vi "GetAreaInfo.vi"(0 "TCP网络连接输入":refnum<k5>, 7 "reference":refnum<vi>, 11 "错误输入（无错误）":errorcluster) -> (8 "值":string[][](array[string]), 15 "错误输出":errorcluster)   [LabVIEW 2014]
uses:
  Global/ClientGlobalCY.vi
panel:
  out "连接的字符串":string
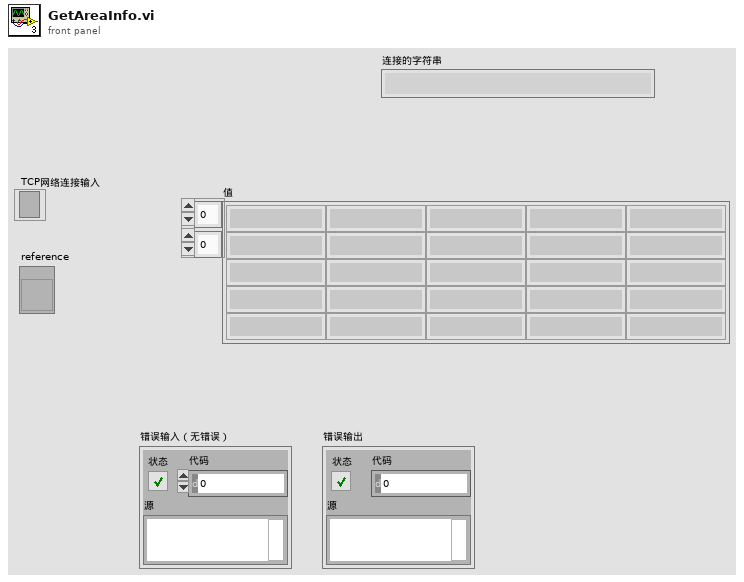
[diagram p1: front panel]
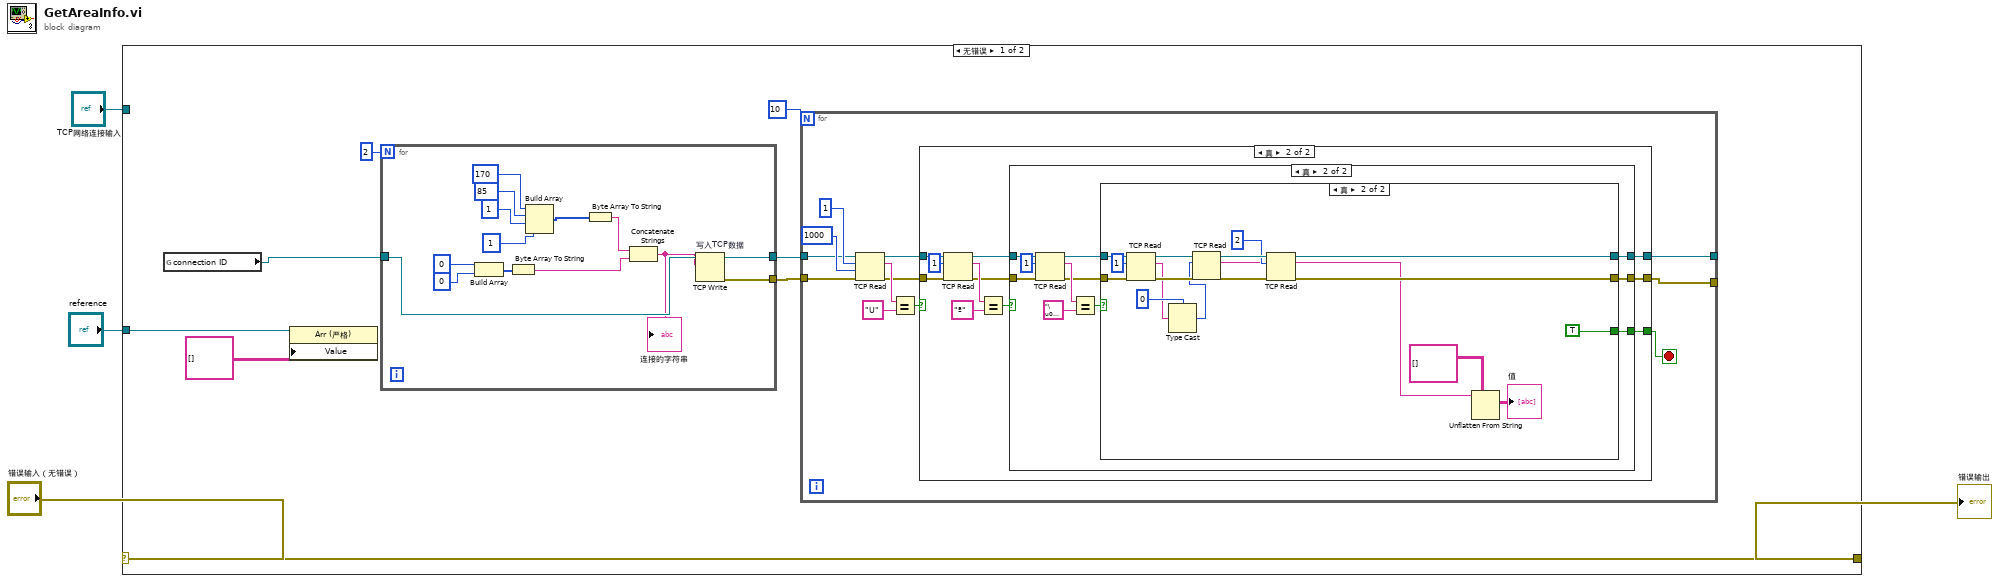
[diagram p0: block diagram]
diagram:
  n1 = case shown="无错误" "错误输入（无错误）" {
    selector: "错误输入（无错误）" -> [w12 w84]
    tunnel: [w12 w84] -> w4
    tunnel: "TCP网络连接输入" -> [_ _]
    tunnel: "reference" -> [w7 _]
    frame No Error {
      n2 = global read "ClientGlobalCY.vi" "connection ID"() -> (w5:refnum<k5>)
      n3 = property class="Arr (严格)"(reference=w7, "Value"=string[][] [] ("值")) -> ()  [unwired: 1 in, 2 out]
      n4 = for {
        N: 2 -> [_]
        tunnel: [w25] -> w10
        tunnel: w5 -> [w24]
        tunnel: [w26] -> w11
        n5 = Build Array(u8 0, u8 0) -> (w17:u8[])
        n6 = Byte Array To String(unsigned byte array=w17) -> (string=w13:string)
        n7 = Build Array(u8 170, u8 85, u8 1, u8 1) -> (w20:u8[])
        n8 = Byte Array To String(unsigned byte array=w20) -> (string=w16:string)
        n9 = Concatenate Strings(w16, w13) -> (w15:string)
        "连接的字符串" <- w15
        n10 = TCP Write "写入TCP数据"(connection ID=w24, data in=w15) -> (connection ID out=w26:refnum<k5>, error out=w25:errorcluster)  [unwired: 2 in, 1 out]
      }
      n11 = for "For循环" {
        N: 10 -> [_]
        tunnel: w11 -> [w31]
        tunnel: w10 -> [w30]
        tunnel: [w28] -> _
        tunnel: [w27] -> _
        stop <- w29 stop-if-true
        n12 = TCP Read(connection ID=w31, bytes to read=1 ("读取的字节"), error in (no error)=w30, 9:1000 ("超时毫秒(25000)")) -> (connection ID out=w34:refnum<k5>, data out=w36:string, error out=w33:errorcluster)  [unwired: 1 in]
        n13 = Equal?(x=w36, y="U") -> (x = y?=w35:bool)
        n14 = case shown="真" w35 {
          tunnel: w34 -> [w40 w48]
          tunnel: w33 -> [w39 w47]
          tunnel: [w40 w43] -> w28
          tunnel: [w39 w42] -> w27
          tunnel: [_ w41] -> w29
          frame False {
          }
          frame True {
            n15 = TCP Read(connection ID=w48, bytes to read=1 ("读取的字节"), error in (no error)=w47) -> (connection ID out=w45:refnum<k5>, data out=w49:string, error out=w44:errorcluster)  [unwired: 2 in]
            n16 = Equal?(x=w49, y="ª") -> (x = y?=w46:bool)
            n17 = case shown="真" w46 {
              tunnel: w45 -> [w53 w61]
              tunnel: w44 -> [w52 w60]
              tunnel: [w53 w56] -> w43
              tunnel: [w52 w55] -> w42
              tunnel: [_ w54] -> w41
              frame False {
              }
              frame True {
                n18 = TCP Read(connection ID=w61, bytes to read=1 ("读取的字节"), error in (no error)=w60) -> (connection ID out=w59:refnum<k5>, data out=w62:string, error out=w58:errorcluster)  [unwired: 2 in]
                n19 = Equal?(x=w62, y="\u0001") -> (x = y?=w57:bool)
                n20 = case shown="真" w57 {
                  tunnel: w59 -> [w66 w82]
                  tunnel: w58 -> [w65 w81]
                  tunnel: [w66 w73] -> w56
                  tunnel: [w65 w74] -> w55
                  tunnel: [_ TRUE] -> w54
                  frame False {
                  }
                  frame True {
                    n21 = TCP Read(connection ID=w82, bytes to read=1 ("读取的字节"), error in (no error)=w81) -> (connection ID out=w80:refnum<k5>, data out=w70:string, error out=w79:errorcluster)  [unwired: 2 in]
                    n22 = Type Cast(type=u8 0, x=w70) -> (*(type *) &x=w71:u8)
                    n23 = TCP Read(connection ID=w80, bytes to read=w71, error in (no error)=w79) -> (connection ID out=w76:refnum<k5>, data out=w69:string, error out=w75:errorcluster)  [unwired: 2 in]
                    n24 = TCP Read(connection ID=w76, bytes to read=2 ("读取的字节"), error in (no error)=w75) -> (connection ID out=w73:refnum<k5>, error out=w74:errorcluster)  [unwired: 2 in, 1 out]
                    n25 = Unflatten From String(type=string[][] [], binary string=w69) -> (value=→"值":string[][])  [unwired: 3 in, 2 out]
                  }
                }
              }
            }
          }
        }
      }
    }
    frame Error {
    }
  }
  "错误输出" <- w4
